vi "Measure Text.vi"(5 "Encoding":refnum<k24>, 7 "Font":refnum<k24>, 8 "error in (no error)":errorcluster, 10 "Text Raw":u8[](array[numeric]), 11 "Canvas in":refnum<class "Drawer .Net.lvclass">) -> (0 "error out":errorcluster, 1 "Size":cluster{"Width":sgl, "Height":sgl}, 2 "Text Raw":u8[](array[numeric]), 3 "Canvas out":refnum<class "Drawer .Net.lvclass">)   [LabVIEW 2023, in "Glyph .NET.lvlib" / "Drawer .Net.lvclass"]
uses:
  Drawer .Net.lvclass
  E:/Labview/LV 2023/Libs/LV Symbol/Canvas/LVFont.dll
  LVFont.dll
  System.Drawing
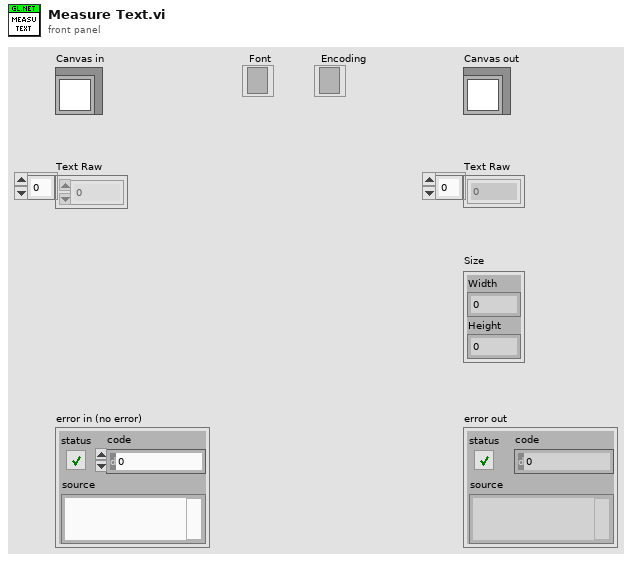
[diagram p1: front panel]
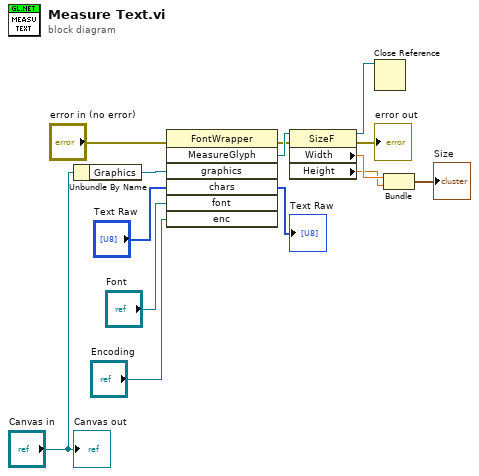
[diagram p0: block diagram]
diagram:
  n1 = Unbundle By Name("Canvas in") -> ("Graphics"=w5:refnum<k24>)
  n2 = invoke class="FontWrapper" method="MeasureGlyph"(error in="error in (no error)", "graphics"=w5, "chars"="Text Raw", "font"="Font", "enc"="Encoding") -> (error out=w10:errorcluster, "MeasureGlyph"=w13:refnum<k24>, "chars"=→"Text Raw":u8[])  [unwired: 2 in, 4 out]
  n3 = property class="SizeF"(reference=w13, error in=w10) -> (reference out=w4:refnum<k24>, error out=→"error out":errorcluster, "Width"=w2:sgl, "Height"=w1:sgl)
  n4 = Close Reference(reference=w4) -> ()  [unwired: 1 in, 1 out]
  n5 = Bundle("Width"=w2, "Height"=w1) -> (→"Size":cluster{"Width":sgl, "Height":sgl})  [unwired: 1 in]
  "Canvas out" <- "Canvas in"
